vi "Close Text File Handle.vi"(8 "error in (no error)":errorcluster, 11 "Byte Stream File in":refnum<file>) -> ()   [LabVIEW 2015]
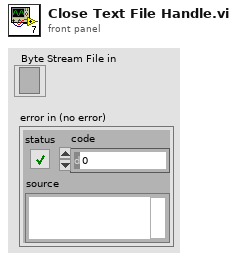
[diagram p1: front panel]
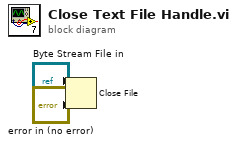
[diagram p0: block diagram]
diagram:
  n1 = Close File(refnum="Byte Stream File in", error in="error in (no error)") -> ()  [unwired: 2 out]
